vi "Write IDN.vi"(8 "error in (no error)":errorcluster, 11 "Instrument in":refnum<class "Instrument.lvclass">) -> (0 "error out":errorcluster, 3 "Instrument out":refnum<class "Instrument.lvclass">)   [LabVIEW 2019, in "Instrument.lvclass"]
doc: "Set the <b>IDN</b> data field:\n- <b>vendor</b> and <b>model</b> are set by overrriding <b>Get SMO Name.vi</b>\n- <b>serial</b> is set at runtime, typically by querying any hardware you are controlling\n- <b>firmware</b> refers to the version of your application, set by ..."
uses:
  Instrument.lvclass
  Instrument.lvclass/Instrument.ctl
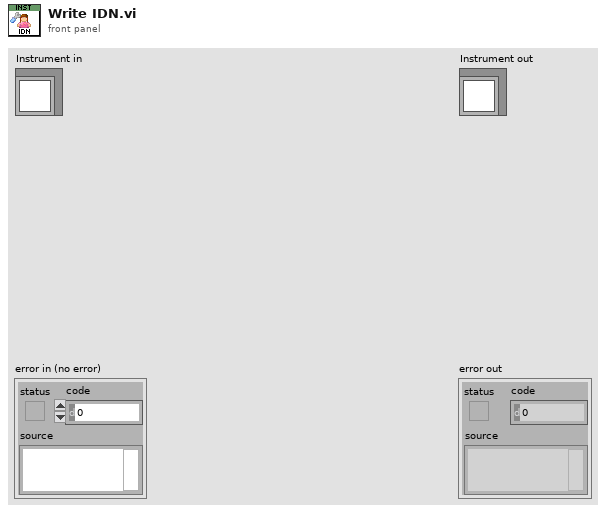
[diagram p1: front panel]
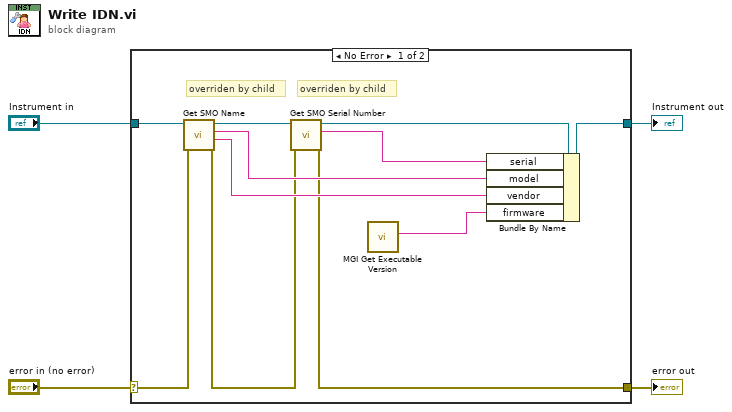
[diagram p0: block diagram]
diagram:
  n1 = case shown="No Error" "error in (no error)" {
    selector: "error in (no error)" -> [w13 w17]
    tunnel: [w6 w17] -> w3
    tunnel: [w15 w16] -> w1
    tunnel: "Instrument in" -> [w14 w16]
    frame No Error {
      # "overriden by child"
      # "overriden by child"
      n2 = call-dynamic "Get SMO Name.vi"("error in (no error)"=w13, "Instrument in"=w14) -> ("error out"=w7:errorcluster, "SMO Vendor"=w12:string, "SMO Name"=w11:string, "Instrument out"=w9:refnum<class "Instrument.lvclass">)  [unwired: 6 in]
      n3 = call-dynamic "Get SMO Serial Number.vi"("error in (no error)"=w7, "Instrument in"=w9) -> ("error out"=w6:errorcluster, "Serial Number"=w5:string, "Instrument out"=w8:refnum<class "Instrument.lvclass">)  [unwired: 7 in]
      n4 = call <userlib>:"MGI Get Executable Version.vi"() -> ("Version"=w10:string)  [unwired: 7 in]
      n5 = Bundle By Name(cluster=w8, "serial"=w5, "model"=w11, "vendor"=w12, "firmware"=w10) -> (w15:refnum<class "Instrument.lvclass">)
    }
    frame Error {
    }
  }
  "error out" <- w3
  "Instrument out" <- w1
